vi "Create RYB Hybrid Color Scale Array.vi"(11 "Include All Colors? (T)":bool=TRUE) -> (2 "RYB Must Include":u32[](array[colorbox])=[16711680, 16776960, 65280, 65535, 255, 16711935], 3 "RYB Array":u32[](array[colorbox]))   [LabVIEW 2015, in "ColorSelector.lvclass"]
doc: "This VI creates the a hybrid Red-Yellow-Blue (RYB) Color Scale Array. It contains the RGB version of Red (FF0000), Yellow (FFFF00), and Blue (0000FF) and adds the color Purple (800080) into the main array. It then realigns the color wheel (Hue in degrees 0-360) for this array. There is the option of whether to leave Cyan (00FFFF) and Magenta (FF00FF) in this array or leave it out.\n<b> </b> <b> </b>\n©2017 Q Software Innovations, LLC (QSI)\nwritten by Quentin Alldredge\nproduced in LabVIEW 2015\n\nsupport@qsoftwareinnovations.com\nwww.qsoftwareinnovations.com\n\nAll rights reserved.\n\nRedistribution and use in source and binary forms, with or without modification, are permitted provided that the following conditions are met:\n\n * Redistributions of source code must retain the above copyright notice, this list of conditions and the following disclaimer.\n * Redistributions in binary form must reproduce the above copyright notice, this list of conditions and the following disclaimer in the documentation and/or other materials provided with the distribution.\n * Neither the name of Q Software Innovations, LLC. nor the names of its contributors may be used to endorse or promote products derived from this software without specific prior written permission.\n\nTHIS SOFTWARE IS PROVIDED BY THE COPYRIGHT HOLDERS AND CONTRIBUTORS \"AS IS\" AND ANY EXPRESS OR IMPLIED WARRANTIES, INCLUDING, BUT NOT LIMITED TO, THE IMPLIED WARRANTIES OF MERCHANTABILITY AND FITNESS FOR A PARTICULAR PURPOSE ARE DISCLAIMED. IN NO EVENT SHALL THE COPYRIGHT OWNER OR CONTRIBUTORS BE LIABLE FOR ANY DIRECT, INDIRECT, INCIDENTAL, SPECIAL, EXEMPLARY, OR CONSEQUENTIAL DAMAGES (INCLUDING, BUT NOT LIMITED TO, PROCUREMENT OF SUBSTITUTE GOODS OR SERVICES; LOSS OF USE, DATA, OR PROFITS; OR BUSINESS INTERRUPTION) HOWEVER CAUSED AND ON ANY THEORY OF LIABILITY, WHETHER IN CONTRACT, STRICT LIABILITY, OR TORT (INCLUDING NEGLIGENCE OR OTHERWISE) ARISING IN ANY WAY OUT OF THE USE OF THIS SOFTWARE, EVEN IF ADVISED OF THE POSSIBILITY OF SUCH DAMAGE."
uses:
  ColorSelector.lvclass
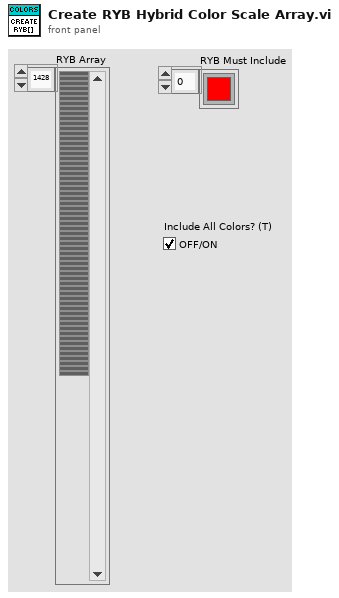
[diagram p1: front panel]
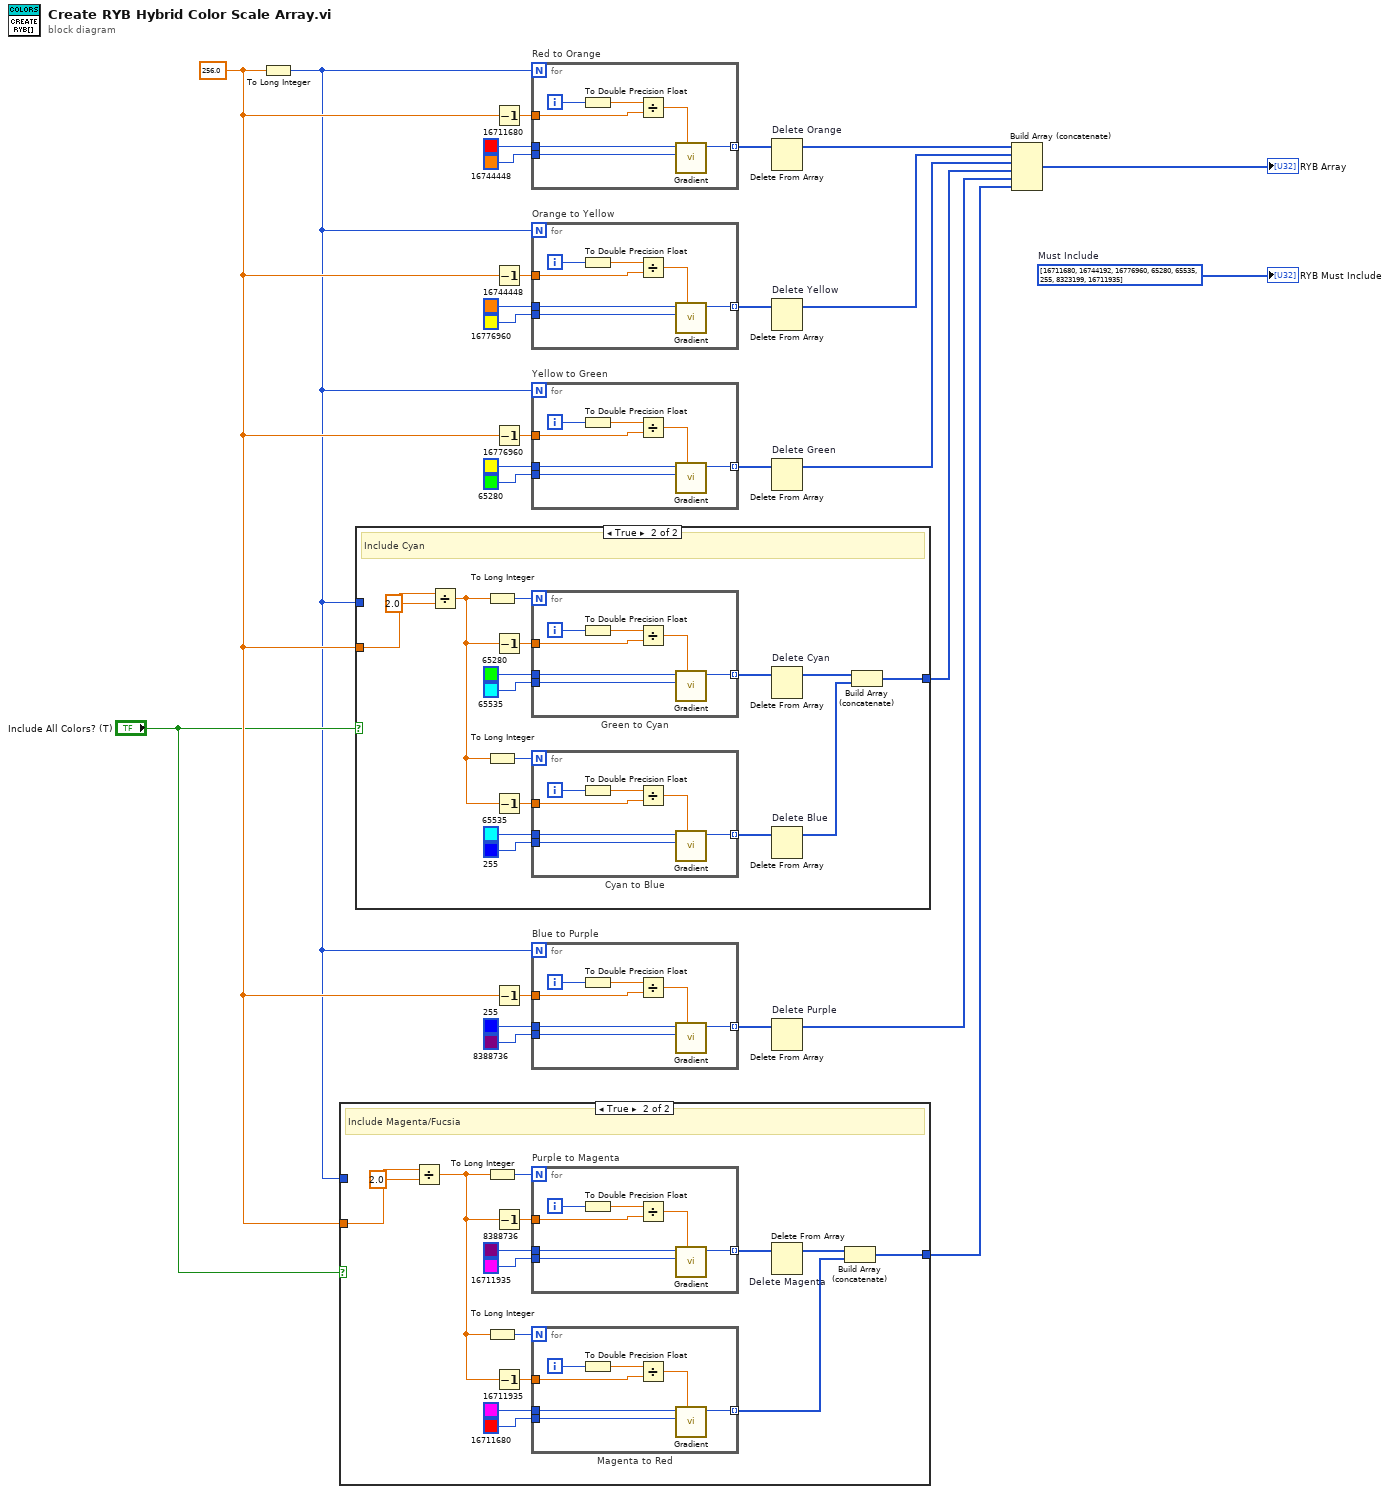
[diagram p0: block diagram]
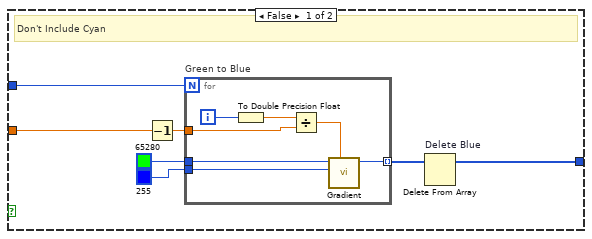
[diagram p2: hidden frame]
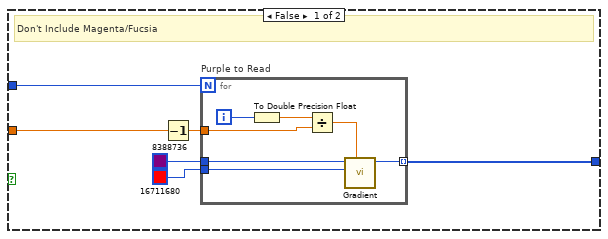
[diagram p3: hidden frame]
diagram:
  w26 = u32[] [16711680, 16744192, 16776960, 65280, 65535, 255, 8323199, 16711935]  # Must Include
  w3 = 256.0
  n1 = To Long Integer(number=w3) -> (32bit integer=w1:i32)
  n2 = case shown="True" "Include All Colors? (T)" {
    tunnel: w3 -> [w28 w44]
    tunnel: [w31 w42] -> w4
    tunnel: w1 -> [w29 _]
    frame False {
      # "Don't Include Magenta/Fucsia"
      n3 = Decrement(x=w28) -> (x-1=w30:dbl)
      n4 = for "Purple to Read" {
        N: w29 -> [_]
        tunnel: [w34] -> w31 mode=indexing
        tunnel: u32 8388736 -> [w40]
        tunnel: u32 16711680 -> [w39]
        tunnel: w30 -> [w35]
        i -> [w37]
        n5 = To Double Precision Float(number=w37) -> (double precision float=w38:dbl)
        n6 = Divide(x=w38, y=w35) -> (x/y=w36:dbl)
        n7 = call "Gradient.vi"("Percent"=w36, "End Color"=w39, "Start Color"=w40) -> ("Gradient Color"=w34:u32)  [unwired: 8 in]
      }
    }
    frame True {
      # "Include Magenta/Fucsia"
      n8 = Divide(x=w44, y=2.0) -> (x/y=w43:dbl)
      n9 = To Long Integer(number=w43) -> (32bit integer=w51:i32)
      n10 = To Long Integer(number=w43) -> (32bit integer=w52:i32)
      n11 = Decrement(x=w43) -> (x-1=w47:dbl)
      n12 = Decrement(x=w43) -> (x-1=w55:dbl)
      n13 = for "Purple to Magenta" {
        N: w51 -> [_]
        tunnel: [w56] -> w48 mode=indexing
        tunnel: u32 8388736 -> [w62]
        tunnel: u32 16711935 -> [w61]
        tunnel: w47 -> [w57]
        i -> [w59]
        n14 = To Double Precision Float(number=w59) -> (double precision float=w60:dbl)
        n15 = Divide(x=w60, y=w57) -> (x/y=w58:dbl)
        n16 = call "Gradient.vi"("Percent"=w58, "End Color"=w61, "Start Color"=w62) -> ("Gradient Color"=w56:u32)  [unwired: 8 in]
      }
      n17 = for "Magenta to Red" {
        N: w52 -> [_]
        tunnel: [w63] -> w41 mode=indexing
        tunnel: u32 16711935 -> [w69]
        tunnel: u32 16711680 -> [w68]
        tunnel: w55 -> [w64]
        i -> [w66]
        n18 = To Double Precision Float(number=w66) -> (double precision float=w67:dbl)
        n19 = Divide(x=w67, y=w64) -> (x/y=w65:dbl)
        n20 = call "Gradient.vi"("Percent"=w65, "End Color"=w68, "Start Color"=w69) -> ("Gradient Color"=w63:u32)  [unwired: 8 in]
      }
      n21 = Delete From Array "Delete Magenta"(array=w48) -> (array with subset deleted=w46:u32[])  [unwired: 2 in, 1 out]
      n22 = Build Array (concatenate)(w46, w41) -> (w42:u32[])
    }
  }
  n23 = case shown="True" "Include All Colors? (T)" {
    tunnel: [w71 w88] -> w10
    tunnel: w1 -> [w72 _]
    tunnel: w3 -> [w70 w85]
    frame False {
      # "Don't Include Cyan"
      n24 = Decrement(x=w70) -> (x-1=w76:dbl)
      n25 = for "Green to Blue" {
        N: w72 -> [_]
        tunnel: [w77] -> w75 mode=indexing
        tunnel: u32 65280 -> [w83]
        tunnel: u32 255 -> [w82]
        tunnel: w76 -> [w78]
        i -> [w80]
        n26 = To Double Precision Float(number=w80) -> (double precision float=w81:dbl)
        n27 = Divide(x=w81, y=w78) -> (x/y=w79:dbl)
        n28 = call "Gradient.vi"("Percent"=w79, "End Color"=w82, "Start Color"=w83) -> ("Gradient Color"=w77:u32)  [unwired: 8 in]
      }
      n29 = Delete From Array "Delete Blue"(array=w75) -> (array with subset deleted=w71:u32[])  [unwired: 2 in, 1 out]
    }
    frame True {
      # "Include Cyan"
      n30 = Divide(x=w85, y=2.0) -> (x/y=w84:dbl)
      n31 = To Long Integer(number=w84) -> (32bit integer=w95:i32)
      n32 = To Long Integer(number=w84) -> (32bit integer=w93:i32)
      n33 = Decrement(x=w84) -> (x-1=w99:dbl)
      n34 = Decrement(x=w84) -> (x-1=w89:dbl)
      n35 = for "Green to Cyan" {
        N: w95 -> [_]
        tunnel: [w100] -> w98 mode=indexing
        tunnel: u32 65280 -> [w106]
        tunnel: u32 65535 -> [w105]
        tunnel: w99 -> [w101]
        i -> [w103]
        n36 = To Double Precision Float(number=w103) -> (double precision float=w104:dbl)
        n37 = Divide(x=w104, y=w101) -> (x/y=w102:dbl)
        n38 = call "Gradient.vi"("Percent"=w102, "End Color"=w105, "Start Color"=w106) -> ("Gradient Color"=w100:u32)  [unwired: 8 in]
      }
      n39 = for "Cyan to Blue" {
        N: w93 -> [_]
        tunnel: [w107] -> w90 mode=indexing
        tunnel: u32 65535 -> [w113]
        tunnel: u32 255 -> [w112]
        tunnel: w89 -> [w108]
        i -> [w110]
        n40 = To Double Precision Float(number=w110) -> (double precision float=w111:dbl)
        n41 = Divide(x=w111, y=w108) -> (x/y=w109:dbl)
        n42 = call "Gradient.vi"("Percent"=w109, "End Color"=w112, "Start Color"=w113) -> ("Gradient Color"=w107:u32)  [unwired: 8 in]
      }
      n43 = Delete From Array "Delete Cyan"(array=w98) -> (array with subset deleted=w94:u32[])  [unwired: 2 in, 1 out]
      n44 = Delete From Array "Delete Blue"(array=w90) -> (array with subset deleted=w87:u32[])  [unwired: 2 in, 1 out]
      n45 = Build Array (concatenate)(w94, w87) -> (w88:u32[])
    }
  }
  n46 = Decrement(x=w3) -> (x-1=w21:dbl)
  n47 = Decrement(x=w3) -> (x-1=w20:dbl)
  n48 = Decrement(x=w3) -> (x-1=w12:dbl)
  n49 = Decrement(x=w3) -> (x-1=w9:dbl)
  n50 = for "Red to Orange" {
    N: w1 -> [_]
    tunnel: [w114] -> w25 mode=indexing
    tunnel: u32 16711680 -> [w120]
    tunnel: u32 16744448 -> [w119]
    tunnel: w21 -> [w115]
    i -> [w117]
    n51 = To Double Precision Float(number=w117) -> (double precision float=w118:dbl)
    n52 = Divide(x=w118, y=w115) -> (x/y=w116:dbl)
    n53 = call "Gradient.vi"("Percent"=w116, "End Color"=w119, "Start Color"=w120) -> ("Gradient Color"=w114:u32)  [unwired: 8 in]
  }
  n54 = for "Orange to Yellow" {
    N: w1 -> [_]
    tunnel: [w121] -> w19 mode=indexing
    tunnel: u32 16744448 -> [w127]
    tunnel: u32 16776960 -> [w126]
    tunnel: w20 -> [w122]
    i -> [w124]
    n55 = To Double Precision Float(number=w124) -> (double precision float=w125:dbl)
    n56 = Divide(x=w125, y=w122) -> (x/y=w123:dbl)
    n57 = call "Gradient.vi"("Percent"=w123, "End Color"=w126, "Start Color"=w127) -> ("Gradient Color"=w121:u32)  [unwired: 8 in]
  }
  n58 = for "Yellow to Green" {
    N: w1 -> [_]
    tunnel: [w128] -> w13 mode=indexing
    tunnel: u32 16776960 -> [w134]
    tunnel: u32 65280 -> [w133]
    tunnel: w12 -> [w129]
    i -> [w131]
    n59 = To Double Precision Float(number=w131) -> (double precision float=w132:dbl)
    n60 = Divide(x=w132, y=w129) -> (x/y=w130:dbl)
    n61 = call "Gradient.vi"("Percent"=w130, "End Color"=w133, "Start Color"=w134) -> ("Gradient Color"=w128:u32)  [unwired: 8 in]
  }
  n62 = for "Blue to Purple" {
    N: w1 -> [_]
    tunnel: [w135] -> w8 mode=indexing
    tunnel: u32 255 -> [w141]
    tunnel: u32 8388736 -> [w140]
    tunnel: w9 -> [w136]
    i -> [w138]
    n63 = To Double Precision Float(number=w138) -> (double precision float=w139:dbl)
    n64 = Divide(x=w139, y=w136) -> (x/y=w137:dbl)
    n65 = call "Gradient.vi"("Percent"=w137, "End Color"=w140, "Start Color"=w141) -> ("Gradient Color"=w135:u32)  [unwired: 8 in]
  }
  n66 = Delete From Array "Delete Orange"(array=w25) -> (array with subset deleted=w24:u32[])  [unwired: 2 in, 1 out]
  n67 = Delete From Array "Delete Yellow"(array=w19) -> (array with subset deleted=w16:u32[])  [unwired: 2 in, 1 out]
  n68 = Delete From Array "Delete Green"(array=w13) -> (array with subset deleted=w11:u32[])  [unwired: 2 in, 1 out]
  n69 = Delete From Array "Delete Purple"(array=w8) -> (array with subset deleted=w5:u32[])  [unwired: 2 in, 1 out]
  n70 = Build Array (concatenate)(w24, w16, w11, w10, w5, w4) -> (→"RYB Array":u32[])
  "RYB Must Include" <- w26
